vi "solar_voy Check Voy Header IDs.vi"(8 "error in":errorcluster, 11 "Voyager Refnum":T1) -> (0 "Error out":errorcluster, 3 "Voyager Refnum out":T1)   [LabVIEW 2018]
doc: "This VI is used after registering to check every voyager header id for each command and telemetry item and ensuring there are no duplicates."
uses:
  solar_voy_ctl Voyager Refnum.ctl
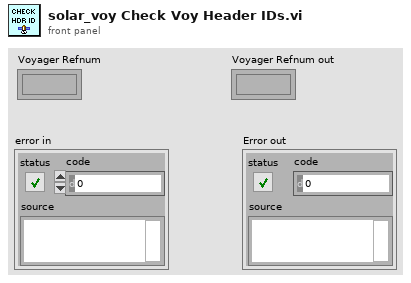
[diagram p1: front panel]
types:
  T1 = typedef "solar_voy_ctl Voyager Refnum.ctl" = refnum<k1>
  T2 = typedef "solar_voy_ctl Voyager.ctl" = cluster{"PACKETS":T3[], "COSMOS_Root":path, "CMD_HDR":T8, "TLM_HDR":T8, "TCPs":T9[], "VoyagerIDOffset":cluster{"VoyagerIDOffset":u16[], "Target Names":string[]}}
  T3 = typedef "solar_voy_def_ctl PACKET.ctl" = cluster{"PACKET_ID":T4, "ENDIAN":enum8{"BIG", "LITTLE"}, "DESC":string, "HZRD":bool, "ITEMS":T5[], "NoExport":bool, "last_time":timestamp, "last_count":u32, "last_data":string}
  T4 = typedef "solar_voy_def_ctl PACKET_ID.ctl" = cluster{"ID":u16, "CMD":enum8{"CMD", "TLM"}, "TARGET":string, "PACKET":string}
  T5 = typedef "solar_voy_def_ctl ITEM.ctl" = cluster{"NAME":string, "OFFSET":i32, "SIZE":i32, "TYPE":T6, "EACH_SIZE":i32, "LVTYPE":T7, "MIN":dbl, "MAX":dbl, "DEFAULT":string, "DESC":string, "ID":bool, "MODIFIERS":variant, "last_value":variant}
  T6 = typedef "solar_voy_def_ctl ITEM TYPE.ctl" = enum8{"BLOCK", "INT", "UINT", "FLOAT", "STRING"}
  T7 = typedef "solar_type Item Type.ctl" = enum16{"NULL", "UNKNOWN", "CLUSTER", "I8", "I16", "I32", "I64", "U8", "U16", "U32", "U64", "U8_ENUM", "U16_ENUM", "U32_ENUM", "SGL", "DBL", "BOOLEAN", "STRING", "PATH", "VISA", "TAG", "TIME", "I8_1D", "I16_1D", "I32_1D", "I64_1D", "U8_1D", "U16_1D", "U32_1D", "U64_1D", "U8_ENUM_1D", "U16_ENUM_1D", "U32_ENUM_1D", "SGL_1D", "DBL_1D", "BOOLEAN_1D", "STRING_1D", "PATH_1D", "VISA_1D", "TAG_1D", "TIME_1D", "I8_2D", "I16_2D", "I32_2D", "I64_2D", "U8_2D", "U16_2D", "U32_2D", "U64_2D", "U8_ENUM_2D", "U16_ENUM_2D", "U32_ENUM_2D", "SGL_2D", "DBL_2D", "BOOLEAN_2D", "STRING_2D", "PATH_2D", "VISA_2D", "TAG_2D", "TIME_2D"}
  T8 = typedef "solar_voy_def_ctl HDR.ctl" = cluster{"ITEMS":T5[], "LENGTH_NAME":string, "LENGTH_VALUE_OFFSET":i32, "ID_NAME":string, "ENDIAN":enum8{"BIG", "LITTLE"}, "GUID_NAME":string, "DEFAULT_TARGET":string, "DEFAULT_PACKET":string, "DEFAULT_ERROR":string}
  T9 = typedef "solar_voy_ctl TCP.ctl" = cluster{"Connected":bool, "Port":u16, "Listener":refnum<k5>, "ServerIP":string, "TCP":refnum<k5>, "Setup":T10, "VIRefnum":refnum<vi>, "TARGETS_CMD":string[], "TARGETS_TLM":string[]}
  T10 = typedef "solar_voy_ctl Port Setup.ctl" = enum8{"SERVER", "CLIENT", "SERVER_CMD", "SERVER_TLM"}
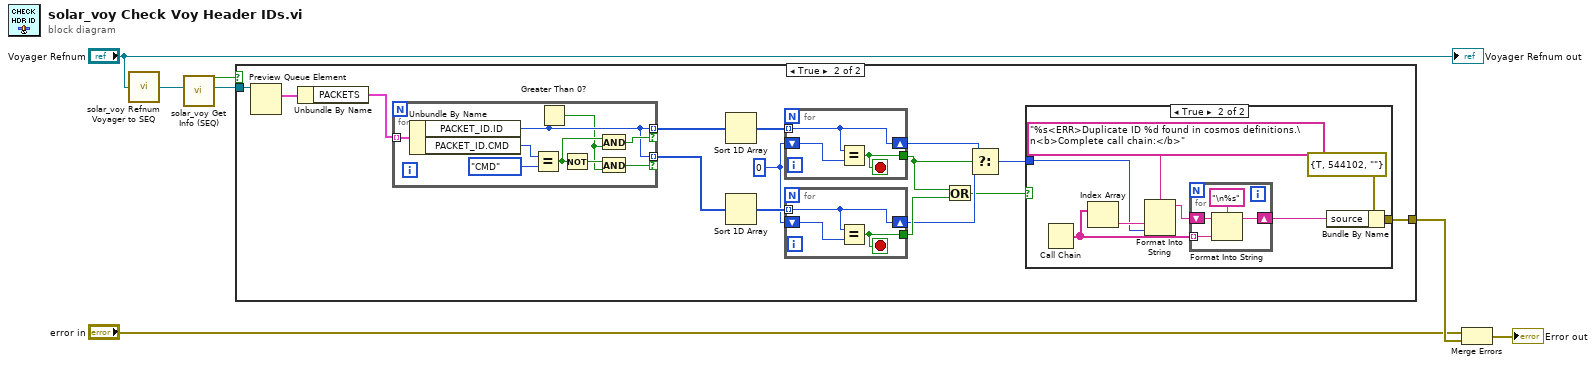
[diagram p0: block diagram]
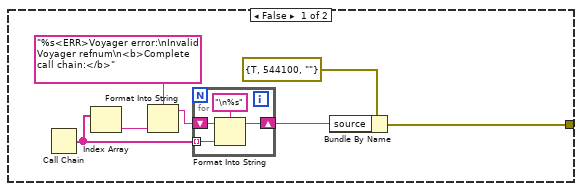
[diagram p2: hidden frame]
diagram:
  n1 = call "solar_voy Refnum Voyager to SEQ.vi"("Voyager Refnum"="Voyager Refnum") -> ("Voyager SEQ"=w7:refnum<queue>)
  n2 = call "solar_voy Get Info (SEQ).vi"("Voyager SEQ in"=w7) -> ("Voyager SEQ out"=w5:refnum<queue>, "Valid?"=w6:bool)  [unwired: 8 in, 1 out]
  n3 = case shown="True" w6 {
    tunnel: w5 -> [_ w22]
    tunnel: [w8 w19] -> w3
    frame False {
      n4 = Call Chain() -> (call chain=w11:string[])
      n5 = Index Array(array=w11) -> (element=w13:string)  [unwired: 1 in]
      n6 = Format Into String(format string="%s<ERR>Voyager error:\nInvalid Voyager refnum\n<b>Complete call chain:</b>", w13) -> (resulting string=w12:string)  [unwired: 2 in, 1 out]
      n7 = for {
        tunnel: w11 -> [w18] mode=indexing
        shift-right: [w17] -> w10
        shift-left: w12 -> [w16]
        n8 = Format Into String(format string="\n%s", initial string=w16, w18) -> (resulting string=w17:string)  [unwired: 1 in, 1 out]
      }
      n9 = Bundle By Name(cluster=errorcluster {"status"=TRUE, "code"=544100, "source"=""} ("error in (no error)"), "source"=w10) -> (w8:errorcluster)
    }
    frame True {
      w25 = u16 0
      n10 = Preview Queue Element(queue=w22) -> (element=w21:T2)  [unwired: 2 in, 3 out]
      n11 = Unbundle By Name(w21) -> ("PACKETS"=w20:T3[])
      n12 = for {
        tunnel: w20 -> [w39] mode=indexing
        tunnel: [w35] -> w24 mode=indexing if=w36
        tunnel: [w35] -> w23 mode=indexing if=w37
        n13 = Unbundle By Name(w39) -> ("PACKET_ID.ID"=w35:u16, "PACKET_ID.CMD"=w42:enum8{"CMD", "TLM"})
        n14 = Equal?(x=w42, y=enum8{"CMD", "TLM"}."CMD") -> (x = y?=w40:bool)
        n15 = Greater Than 0?(x=w35) -> (x > 0?=w34:bool)
        n16 = Not(x=w40) -> (.not. x?=w38:bool)
        n17 = And(x=w40, y=w34) -> (x .and. y?=w36:bool)
        n18 = And(x=w38, y=w34) -> (x .and. y?=w37:bool)
      }
      n19 = Sort 1D Array(array=w24) -> (sorted array=w33:u16[])
      n20 = Sort 1D Array(array=w23) -> (sorted array=w32:u16[])
      n21 = for {
        tunnel: w33 -> [w60] mode=indexing
        shift-right: [w60] -> w29
        shift-left: w25 -> [w59]
        tunnel: [w58] -> w30
        stop <- w58 stop-if-true
        n22 = Equal?(x=w60, y=w59) -> (x = y?=w58:bool)
      }
      n23 = for {
        tunnel: w32 -> [w57] mode=indexing
        shift-right: [w57] -> w28
        shift-left: w25 -> [w56]
        tunnel: [w55] -> w31
        stop <- w55 stop-if-true
        n24 = Equal?(x=w57, y=w56) -> (x = y?=w55:bool)
      }
      n25 = Or(x=w30, y=w31) -> (x .or. y?=w26:bool)
      n26 = Select(t=w29, s=w30, f=w28) -> (s? t:f=w27:u16)
      n27 = case shown="True" w26 {
        tunnel: w27 -> [_ w44]
        tunnel: [_ w43] -> w19
        frame False {
        }
        frame True {
          n28 = Call Chain() -> (call chain=w48:string[])
          n29 = Index Array(array=w48) -> (element=w46:string)  [unwired: 1 in]
          n30 = Format Into String(format string="%s<ERR>Duplicate ID %d found in cosmos definitions.\n<b>Complete call chain:</b>", w46, w44) -> (resulting string=w47:string)  [unwired: 2 in, 1 out]
          n31 = for {
            tunnel: w48 -> [w54] mode=indexing
            shift-right: [w53] -> w49
            shift-left: w47 -> [w52]
            n32 = Format Into String(format string="\n%s", initial string=w52, w54) -> (resulting string=w53:string)  [unwired: 1 in, 1 out]
          }
          n33 = Bundle By Name(cluster=errorcluster {"status"=TRUE, "code"=544102, "source"=""} ("error in (no error)"), "source"=w49) -> (w43:errorcluster)
        }
      }
    }
  }
  n34 = Merge Errors("error in", w3) -> (→"Error out":errorcluster)
  "Voyager Refnum out" <- "Voyager Refnum"
